vi "Intake Controller.vi"(8 "error in":errorcluster) -> ()   [LabVIEW 2017]
doc: "This VI executes continuously carrying out the current operation and responding to updates or new operations. It will often contain the timing or control code that is difficult to place directly in TeleOp. This VI generally opens all sensors and motors and isolates the rest of the robot code from knowing how the operations are carried out."
uses:
  <vilib>/Rock Robotics/WPI/Framework/Completion Status.ctl
  Intake Setpoints.ctl
  Intake Operations.ctl
  <vilib>/Rock Robotics/SystemInterfaces/DIO/FPGA_DIOPWMChannel.ctl
  <vilib>/Rock Robotics/SystemInterfaces/DIO/FPGA_DIOChannel.ctl
  <extravilib>/ChannelInstances/Lossy Stream-bool/Write With Abort.vi
  <extravilib>/ChannelInstances/Lossy Stream-bool/Read With Abort.vi
  <extravilib>/ChannelInstances/Lossy Stream-bool/Endpoint.vi
  <extravilib>/ChannelInstances/Lossy Stream-bool/EndpointRead.vi
  <vilib>/Rock Robotics/WPI/RobotDrive/WPI_RobotDriveOpen2MotorWithSPARK.vi
  <vilib>/Rock Robotics/WPI/Ultrasonic/WPI_SonarMB1010DigitalOpen.vi
  <extravilib>/ChannelInstances/Lossy Stream-bool/Instantiate.vi
  Framework/Robot Global Data.vi
  <extravilib>/ChannelInstances/Lossy Stream-bool/)Channel.vi
  <resource>/ChannelSupport/_ChannelSupport/WaitIfNeeded.vi
  <vilib>/Rock Robotics/WPI/Ultrasonic/WPI_SonarMB1010DigitalGetRange.vi
  Intake Published Globals.vi
  <vilib>/Rock Robotics/Network Tables/NT Write Number.vi
  <vilib>/Rock Robotics/Network Tables/NT Write Boolean.vi
  <extravilib>/ChannelInstances/Lossy Stream-bool.lvlib
panel:
  out "Waveform Chart":dbl(graph)=37.89591836734694
  out "Distance":dbl=37.89591836734694
  in  "HasCubeDisance":dbl=9.0
  out "Has Cube":bool
  in  "Interactive Values":T1
  out "Current\nCmd":string="Started at  12:56:38.436\nDefault: Reserve,  S 0.0, D 0.000000"
  in  "Buttons":cluster{"Execute Cmd":bool, "Abort Cmd":bool}
  out "Command Timing":cluster{"Start Time (ms)":u32, "Iterations":i32}={"Start Time (ms)"=8116528, "Iterations"=0}
  out "Status":T3
  # "Tip: It may be helpful to observe inputs and sensor values.\nYou may also want to display tuning or debugging controls."
  # "Interactive Command: You may fill in the settings for a command\nand schedule it with the Execute button. You can observe and abort\nany command while fine tuning the code for the controller."
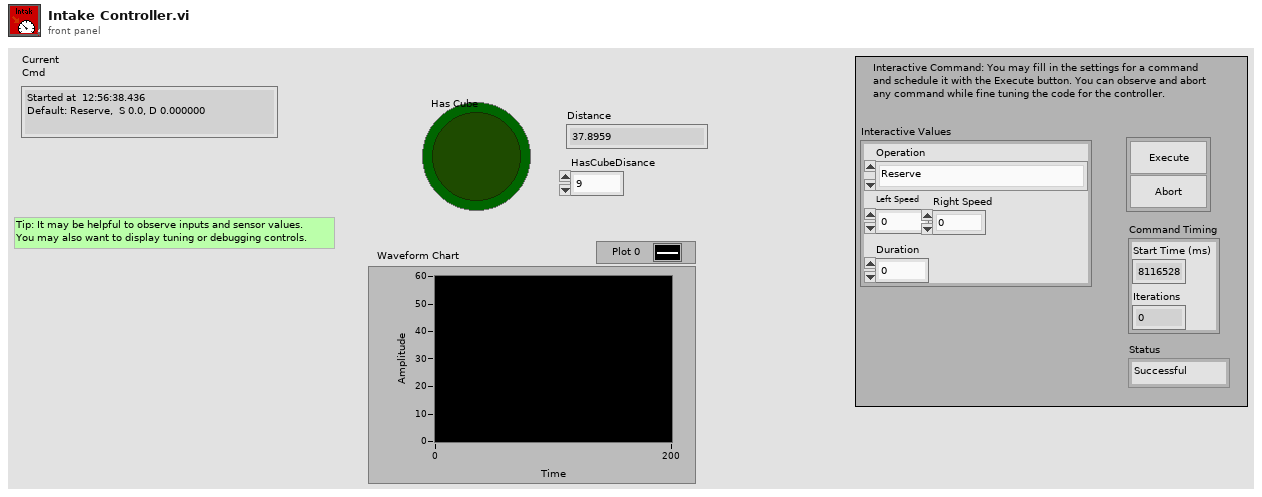
[diagram p1: front panel]
types:
  T1 = typedef "Intake Setpoints.ctl" = cluster{"Operation":T2, "Left Speed":dbl, "Duration":dbl, "Right Speed":dbl}
  T2 = typedef "Intake Operations.ctl" = enum16{"Reserve", "Read Current", "Immediate", "Intake for Duration", "Intake Until Cube"}
  T3 = typedef "Completion Status.ctl" = enum16{"Successful", "Aborted", "Incomplete"}
  T4 = typedef "FPGA_DIOChannel.ctl" = enum8{"DIO 0", "DIO 1", "DIO 2", "DIO 3", "DIO 4", "DIO 5", "DIO 6", "DIO 7", "DIO 8", "DIO 9", "DIO MXP 0", "DIO MXP 1", "DIO MXP 2", "DIO MXP 3", "DIO MXP 4", "DIO MXP 5", "DIO MXP 6", "DIO MXP 7", "DIO MXP 8", "DIO MXP 9", "DIO MXP 10", "DIO MXP 11", "DIO MXP 12", "DIO MXP 13", "DIO MXP 14", "DIO MXP 15", "SPI Port CS1", "SPI Port CS2", "SPI Port CS3", "SPI Port MISO", "SPI Port MOSI", "Invalid"}
  T5 = typedef "FPGA_DIOPWMChannel.ctl" = enum8{"PWM 0", "PWM 1", "PWM 2", "PWM 3", "PWM 4", "PWM 5", "PWM 6", "PWM 7", "PWM 8", "PWM 9", "PWM MXP 0", "PWM MXP 1", "PWM MXP 2", "PWM MXP 3", "PWM MXP 4", "PWM MXP 5", "PWM MXP 6", "PWM MXP 7", "PWM MXP 8", "PWM MXP 9", "Invalid"}
  T6 = typedef "WPI_SonarMB1010DigitalDeviceRef.ctl" = cluster{"CounterDevRef":T7, "Scaling factor (s/in)":dbl}
  T7 = typedef "WPI_CounterDevRef.ctl" = cluster{"DevStatus":errorcluster, "CntIndex":T8}
  T8 = typedef "FPGA_CounterCtrSystemIndex.ctl" = enum8{"Ctr 0", "Ctr 1", "Ctr 2", "Ctr 3", "Ctr 4", "Ctr 5", "Ctr 6", "Ctr 7", "Invalid"}
  T9 = typedef "WPI_RobotDriveDevRef.ctl" = cluster{"DevStatus":errorcluster, "Motors[]":T10[], "Square Inputs":bool, "Max Output":dbl}
  T10 = typedef "WPI_MotorControlDeviceRef.ctl" = cluster{"DeviceStatus":errorcluster, "Type":T11, "PWM":cluster{"PWM Channel":T5, "DeadBand":T12}, "CAN":cluster{"Device Number":u8, "SetOutput VI Ref":variant, "GetOutput VI Ref":variant, "Enable VI Ref":variant, "Disable VI Ref":variant, "Data":variant}, "Invert":bool, "DIO PWM":cluster{"PWM \"Enable\" Channel":T5, "DIOChannel":T4, "PWM Rate":dbl}}
  T11 = typedef "WPI_MotorControlType.ctl" = enum16{"PWM", "CAN", "DIO PWM"}
  T12 = typedef "WPI_PWMDeadband.ctl" = cluster{"Name":string, "maxPositivePwm":i32, "minPositivePwm":i32, "centerPwm":i32, "maxNegativePwm":i32, "minNegativePwm":i32, "angularRange":u16}
  T13 = typedef "Lossy Stream-bool.lvlib/)Channel.ctl" = refnum<queue>
  T14 = typedef "Command Status Info.ctl" = cluster{"Name":string, "Status":T3, "notifier out":T15}
  T15 = typedef "Completion Notifier.ctl" = refnum<notifier>
  T16 = cluster{"Current Command":T1, "Command Timing":cluster{"Start Time (ms)":u32, "Iterations":i32}, "Command Arguments":cluster{"Command Info":T14, "Description":string, "Default Command":T1, "queue out":refnum<queue>, "Subsystem Name":string}}
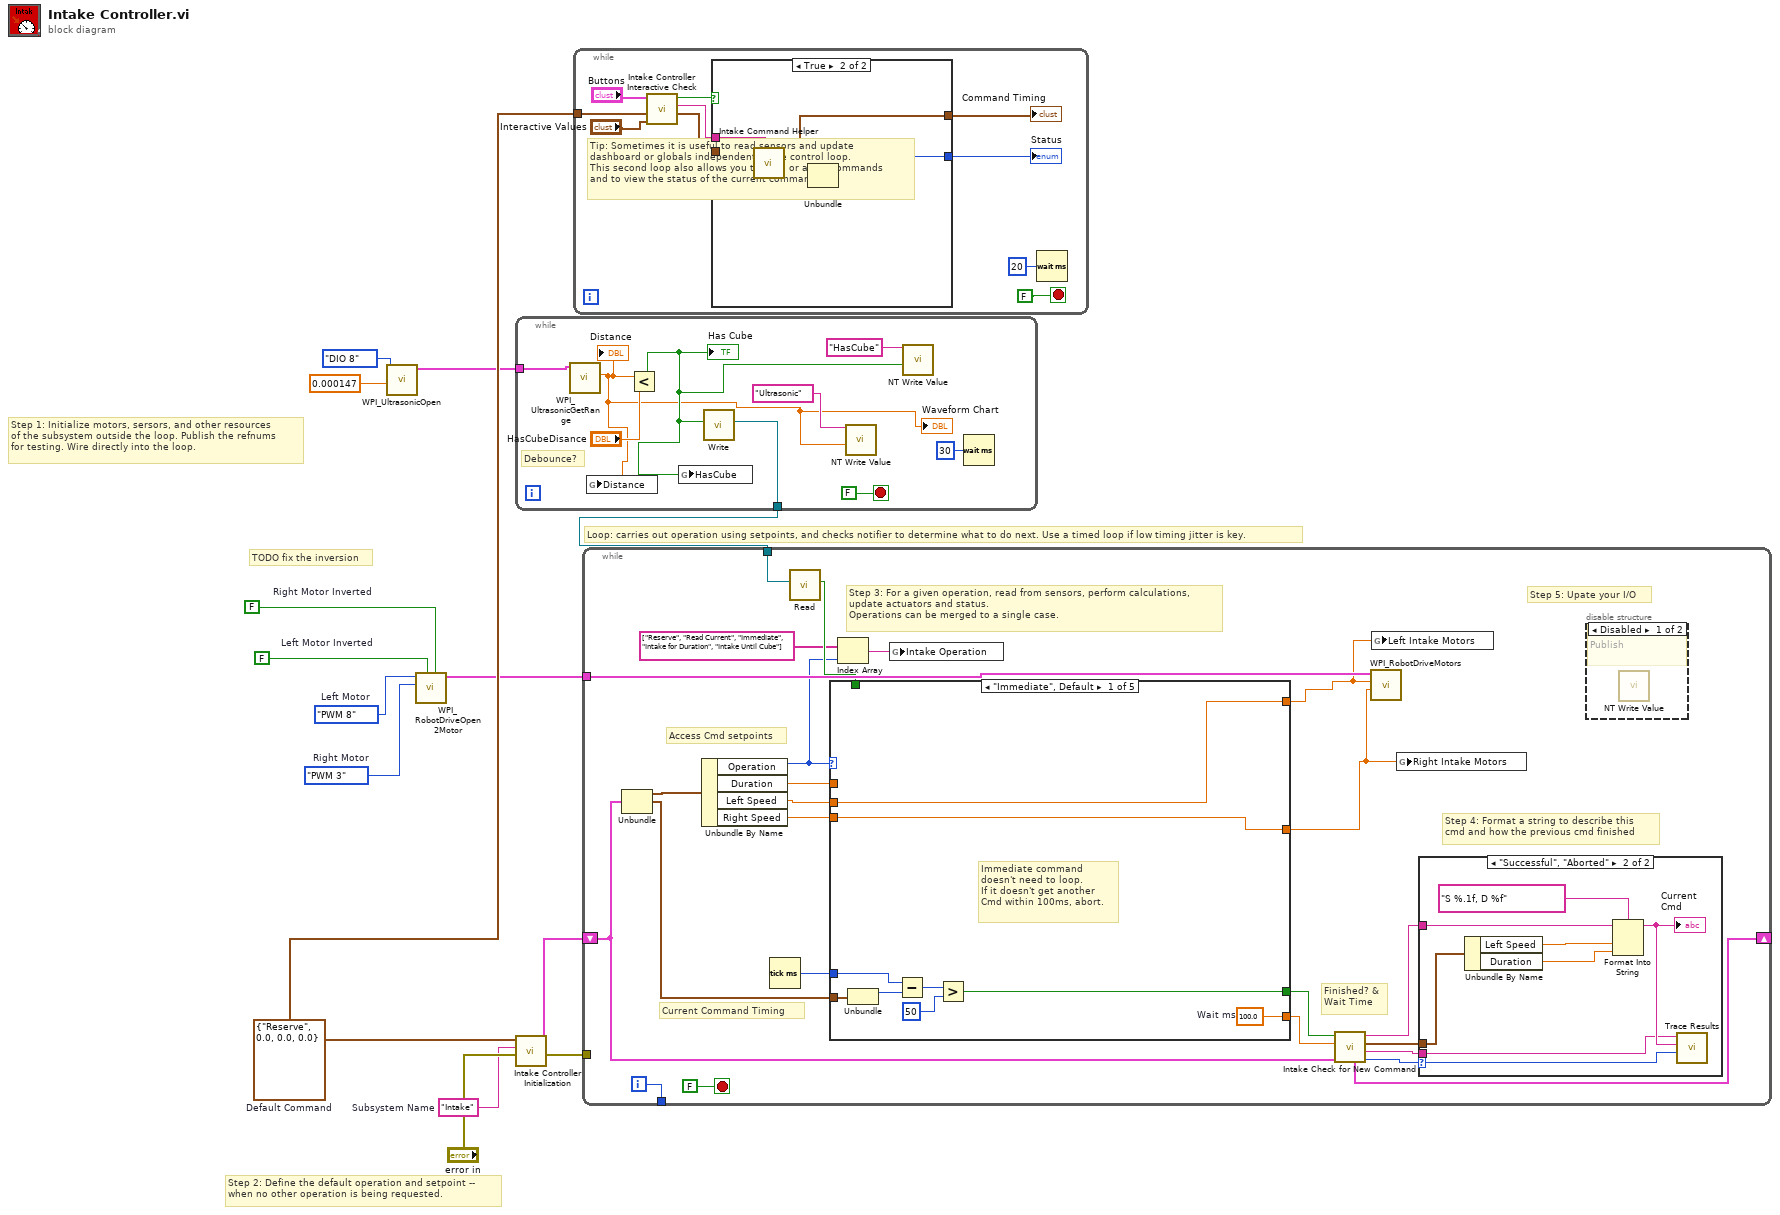
[diagram p0: block diagram]
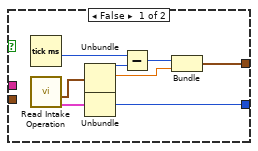
[diagram p2: hidden frame]
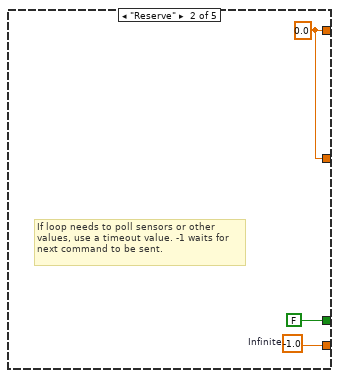
[diagram p3: hidden frame]
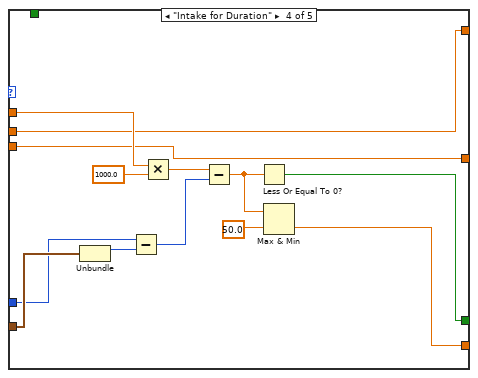
[diagram p5: hidden frame]
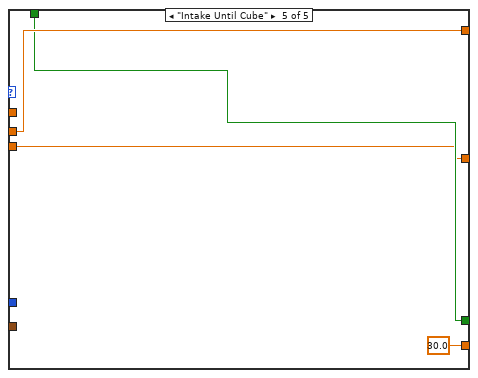
[diagram p6: hidden frame]
diagram:
  w4 = FALSE  # Left Motor Inverted
  w7 = FALSE  # Right Motor Inverted
  w5 = FPGA_DIOPWMChannel."PWM 3"  # Right Motor
  w6 = FPGA_DIOPWMChannel."PWM 8"  # Left Motor
  w10 = T1 {"Operation"=enum."Reserve", "Left Speed"=0.0, "Duration"=0.0, "Right Speed"=0.0}  # Default Command
  w11 = "Intake"  # Subsystem Name
  # "Step 2: Define the default operation and setpoint --\nwhen no other operation is being requested."
  # "TODO fix the inversion"
  # "Tip: Sometimes it is useful to read sensors and update\ndashboard or globals independent of the control loop.\nThis second loop also allows you to send or abort commands\nand to view the status of the current command."
  # "Step 1: Initialize motors, sersors, and other resources\nof the subsystem outside the loop. Publish the refnums\nfor testing. Wire directly into the loop."
  # "Loop: carries out operation using setpoints, and checks notifier to determine what to do next. Use a timed loop if low timing jitter is key."
  n1 = call-poly <vilib>:"WPI_UltrasonicOpen.vi"("Scaling factor (s/in)"=0.000147, "DIO Channel"=FPGA_DIOChannel."DIO 8") -> ("SonarMB1010DigitalDevRef"=w3:T6)  [unwired: 8 in, 1 out]
  n2 = call-poly <vilib>:"WPI_RobotDriveOpen2Motor.vi"("Right Motor Inverted"=w7, "Left Motor Inverted"=w4, "Right Motor"=w5, "Left Motor"=w6) -> ("RobotDriveDevRef"=w8:T9)  [unwired: 6 in, 1 out]
  n3 = while {
    tunnel: w3 -> [w18]
    tunnel: [w21] -> w9
    stop <- FALSE stop-if-true
    # "Debounce?"
    n4 = call-poly <vilib>:"WPI_UltrasonicGetRange.vi"("SonarMB1010DigitalDevRef"=w18) -> ("Distance"=w14:dbl)  [unwired: 8 in, 2 out]
    "Distance" <- w14
    "Waveform Chart" <- w14
    n5 = global write "Intake Published Globals.vi" "Distance"(w14) -> ()
    n6 = Less?(x=w14, y="HasCubeDisance") -> (x < y?=w16:bool)
    "Has Cube" <- w16
    n7 = global write "Intake Published Globals.vi" "HasCube"(w16) -> ()
    n8 = call <extravilib>:"Write.vi"("element"=w16) -> ("channel"=w21:T13)  [unwired: 8 in, 2 out]
    n9 = call-poly <vilib>:"NT Write Value.vi"("Numeric"=w14, "Name"="Ultrasonic") -> ()  [unwired: 9 in, 1 out]
    n10 = call-poly <vilib>:"NT Write Value.vi"("Boolean"=w16, "Name"="HasCube") -> ()  [unwired: 9 in, 1 out]
    n11 = Wait (ms)(milliseconds to wait=u32 30) -> ()  [unwired: 1 out]
  }
  n12 = call "Intake Controller Initialization.vi"("Subsystem Name"=w11, "Default Command"=w10) -> ("Current Command"=w12:T16)  [unwired: 9 in]
  n13 = while {
    tunnel: w10 -> [w29]
    stop <- FALSE stop-if-true
    n14 = call "Intake Controller Interactive Check.vi"("Interactive Command in"="Interactive Values", "Default Command"=w29, "Buttons"="Buttons") -> ("Interactive Command out"=w26:T1, "Trace String"=w27:string, "Schedule"=w28:bool)  [unwired: 6 in]
    n15 = case shown="True" w28 {
      tunnel: [w40 w45] -> w25
      tunnel: w26 -> [_ w43]
      tunnel: [w36 w41] -> w24
      tunnel: w27 -> [_ w44]
      frame False {
        n16 = Tick Count (ms)() -> (millisecond timer value=w35:u32)
        n17 = call "Read Intake Operation.vi"() -> ("Command Info"=w33:T14, "SubSystem Data"=w34:T1)  [unwired: 9 in, 1 out]
        n18 = Unbundle(w34) -> ("Operation"=w39:T2, "Left Speed"=w37:dbl)  [unwired: 2 out]
        n19 = Unbundle(w33) -> ("Status"=w40:T3)  [unwired: 2 out]
        n20 = Subtract(x=w35, y=w39) -> (x-y=w38:u32)
        n21 = Bundle(w38, "Left Speed"=w37) -> (w36:cluster{u32, "Left Speed":dbl})  [unwired: 1 in]
      }
      frame True {
        n22 = call "Intake Command Helper.vi"("Description"=w44, "SubSystem Data"=w43) -> ("Command Info Out"=w42:T14, "Command Timing"=w41:cluster{"Start Time (ms)":u32, "Iterations":i32})  [unwired: 7 in, 1 out]
        n23 = Unbundle(w42) -> ("Status"=w45:T3)  [unwired: 2 out]
      }
    }
    "Status" <- w25
    "Command Timing" <- w24
    n24 = Wait (ms)(milliseconds to wait=u32 20) -> ()  [unwired: 1 out]
  }
  n25 = while {
    shift-right: [w62] -> _
    shift-left: w12 -> [w55]
    tunnel: [w68] -> _
    tunnel: "error in" -> [_]
    tunnel: w8 -> [w54]
    tunnel: w9 -> [w53]
    i -> [w68]
    stop <- FALSE stop-if-true
    # "Step 5: Upate your I/O"
    # "Step 4: Format a string to describe this\ncmd and how the previous cmd finished"
    # "Current Command Timing"
    # "Access Cmd setpoints"
    # "Finished? &\nWait Time"
    # "Step 3: For a given operation, read from sensors, perform calculations,\nupdate actuators and status.\nOperations can be merged to a single case."
    n26 = Unbundle(w55) -> ("Current Command"=w67:T1, "Command Timing"=w64:cluster{"Start Time (ms)":u32, "Iterations":i32})  [unwired: 1 out]
    n27 = Unbundle By Name(w67) -> ("Operation"=w49:T2, "Duration"=w66:dbl, "Left Speed"=w63:dbl, "Right Speed"=w47:dbl)
    n28 = Tick Count (ms)() -> (millisecond timer value=w65:u32)
    n29 = call <extravilib>:"Read.vi"("channel"=w53) -> ("element"=w52:bool)  [unwired: 5 in, 5 out]
    n30 = case shown="\"Immediate\", Default" w49 {
      tunnel: [w78 w81 _ w85 30.0 ("Infinite")] -> w60
      tunnel: [w72 FALSE ("ignore previous (F)") _ w86 w96] -> w61
      tunnel: w64 -> [w74 _ _ w84 _]
      tunnel: w66 -> [_ _ _ w88 _]
      tunnel: w65 -> [w73 _ _ w83 _]
      tunnel: w63 -> [w71 _ _ w87 w98]
      tunnel: [w71 w79 _ w87 w98] -> w51
      tunnel: w52 -> [_ _ _ _ w96]
      tunnel: [w70 w79 _ w82 w95] -> w46
      tunnel: w47 -> [w70 _ _ w82 w95]
      frame "Immediate", Default {
        w78 = 100.0  # Wait ms
        # "Immediate command\ndoesn't need to loop.\nIf it doesn't get another\nCmd within 100ms, abort."
        n31 = Unbundle(w74) -> ("Start Time (ms)"=w77:u32)  [unwired: 1 out]
        n32 = Subtract(x=w73, y=w77) -> (x-y=w76:u32)
        n33 = Greater?(x=w76, y=u8 50 ("Left Motor")) -> (0:w72:bool)
      }
      frame "Reserve" {
        w79 = 0.0 ("Speed")
        w81 = -1.0  # Infinite
        # "If loop needs to poll sensors or other\nvalues, use a timeout value. -1 waits for\nnext command to be sent."
      }
      frame "Read Current" {
      }
      frame "Intake for Duration" {
        n34 = Unbundle(w84) -> ("Start Time (ms)"=w91:u32)  [unwired: 1 out]
        n35 = Subtract(x=w83, y=w91) -> (x-y=w94:u32)
        n36 = Multiply(x=w88, y=1000.0) -> (x*y=w93:dbl)
        n37 = Subtract(x=w93, y=w94) -> (x-y=w90:dbl)
        n38 = Less Or Equal To 0?(x=w90) -> (x <= 0?=w86:bool)
        n39 = Max & Min(x=w90, y=50.0) -> (min(x,y)=w85:dbl)  [unwired: 1 out]
      }
      frame "Intake Until Cube" {
      }
    }
    n40 = Index Array(array=string[] ["Reserve", "Read Current", "Immediate", "Intake for Duration", "Intake Until Cube"] ("Strings []"), index=w49) -> (element=w50:string)
    n41 = global write "Robot Global Data.vi" "Intake Operation"(w50) -> ()
    n42 = call "Intake Check for New Command.vi"("Current Command"=w55, "Wait time (ms)"=w60, "Finished?"=w61) -> ("Completion"=w56:T3, "Subsystem Name"=w57:string, "Current Command"=w58:T1, "Initial Trace String"=w59:string, "NextCommand"=w62:T16)  [unwired: 4 in]
    n43 = call <vilib>:"WPI_RobotDriveMotors.vi"("RightSpeed"=w46, "LeftSpeed"=w51, "RobotDriveDevRef"=w54) -> ()  [unwired: 1 in, 8 out]
    n44 = global write "Robot Global Data.vi" "Left Intake Motors"(w51) -> ()
    n45 = global write "Robot Global Data.vi" "Right Intake Motors"(w46) -> ()
    n46 = case shown="\"Successful\", \"Aborted\"" w56 {
      selector: w56 -> [_ w106]
      tunnel: w59 -> [_ w102]
      tunnel: w58 -> [_ w103]
      tunnel: w57 -> [_ w99]
      frame "Incomplete", Default {
        # "Continuing current command"
      }
      frame "Successful", "Aborted" {
        # "Report and setup for next command"
        n47 = Unbundle By Name(w103) -> ("Left Speed"=w105:dbl, "Duration"=w100:dbl)
        n48 = Format Into String(format string="S %.1f, D %f", initial string=w102, w105, w100) -> (resulting string=w101:string)  [unwired: 1 in, 1 out]
        "Current\nCmd" <- w101
        n49 = call <vilib>:"Trace Results.vi"("Status of previous command"=w106, "Description"=w101, "Subsystem"=w99) -> ()  [unwired: 9 in]
      }
    }
    n50 = disable-structure shown="Disabled" {
      frame Disabled {
        # "Publish"
        n51 = call-poly <vilib>:"NT Write Value.vi"() -> ()  [unwired: 11 in, 1 out]
      }
      frame Enabled {
      }
    }
  }
